vi "DC motor drive with k.vi"() -> ()   [LabVIEW 2019]
uses:
  <vilib>/addons/Control Design/_Model Construction/Data Typedefs.llb/CD Feedback Connections.ctl
  <vilib>/addons/Control Design/_Model Construction/Data Typedefs.llb/CD Root Locus with Gain Info.ctl
  <vilib>/addons/Control Design/_Model Construction/Model Creation.llb/Model Creation SubVI/cd_Create Transfer Function Model.vi
  <vilib>/addons/Control Design/_Utility/Model Viewer.llb/Model Viewer SubVI/cd_Draw Transfer Function Equation (TF).vi
  <vilib>/addons/Control Design/_Model Interconnection/Model Interconnection.llb/Model Interconnection SubVI/cd_Series (TF and TF).vi
  <vilib>/addons/Control Design/_Model Interconnection/Model Interconnection.llb/Model Interconnection SubVI/cd_Matrix Divide Models (TF and TF).vi
  <vilib>/addons/Control Design/_Model Interconnection/Model Interconnection.llb/Model Interconnection SubVI/cd_Feedback (TF and TF).vi
  <vilib>/addons/Control Design/_Model Construction/Special Model Creation.llb/Special Model Creation SubVI/CD Create PID Academic Model.vi
  <vilib>/addons/Control Design/_Model Interconnection/Model Interconnection.llb/Model Interconnection SubVI/cd_Unit Feedback (TF and TF).vi
  <vilib>/addons/Control Design/_Model Conversions/Model Type.llb/Model Conversion SubVI/cd_Convert Transfer Function to Zero-Pole-Gain Model.vi
  <vilib>/addons/Control Design/_Utility/Model Viewer.llb/Model Viewer SubVI/cd_Draw Zero-Pole-Gain Equation (ZPK).vi
  <vilib>/addons/Control Design/_Dynamic Analysis/Dynamic Analysis.llb/Dynamic Analysis subVI/cd_Pole-Zero Map (Transfer Function).vi
  <vilib>/addons/Control Design/_Dynamic Analysis/Dynamic Analysis.llb/Dynamic Analysis subVI/cd_Root Locus (Transfer Function).vi
  <vilib>/addons/Control Design/_Dynamic Analysis/Dynamic Analysis.llb/Dynamic Analysis subVI/cd_Stability (Transfer Function).vi
  <vilib>/addons/Control Design/_Model Construction/NI_LinSys_Model Creation.lvlib
  <vilib>/addons/Control Design/_Utility/NI_CD_Model Viewer.lvlib
  <vilib>/addons/Control Design/_Model Interconnection/NI_CD_Model Interconnection.lvlib
  <vilib>/addons/Control Design/_Dynamic Analysis/NI_CD_Dynamic Analysis.lvlib
  <vilib>/addons/Control Design/_Model Conversions/NI_CD_Model Type.lvlib
  <vilib>/addons/Control Design/_Model Construction/NI_CD_Special Model Creation.lvlib
  <vilib>/addons/Control Design/_Model Construction/NI_LinSys_Data Typedefs.lvlib
panel:
  out "Root Locus Information":T1
  out "Root Locus Graph":cluster{dbl[], dbl[]}[](graph)
  out "Stability":T2(ring)=enum."undetermined"
  out "G9(s)/(G7(s)":picture
  out "Zero-Pole-Gain Model":picture
  out "Overall transfer function":picture
  out "Zeros":cdb[](array[numeric]) format="%.4f"
  out "Poles":cdb[](array[numeric]) format="%.4f"
  out "Pole-Zero Map":cluster{dbl[], dbl[]}[](graph)
  in  "Feedback Connections":T3
  out "G10(s)":picture
  in  "Denominator 10":dbl[](array[numeric]) format="%#.5g"
  in  "Numerator 10":dbl[](array[numeric]) format="%#.5g"
  out "G9(s)":picture
  in  "Denominator 9":dbl[](array[numeric]) format="%#.5g"
  in  "Numerator 9":dbl[](array[numeric]) format="%#.5g"
  out "G8(s)":picture
  in  "Denominator 8":dbl[](array[numeric]) format="%#.5g"
  in  "Numerator 8":dbl[](array[numeric]) format="%#.5g"
  out "G7s)":picture
  in  "Denominator 7":dbl[](array[numeric]) format="%#.5g"
  in  "Numerator 7":dbl[](array[numeric]) format="%#.5g"
  out "G6(s)":picture
  in  "Denominator 6":dbl[](array[numeric]) format="%#.5g"
  in  "Numerator 6":dbl[](array[numeric]) format="%#.5g"
  out "G5(s)":picture
  in  "Denominator 5":dbl[](array[numeric]) format="%#.5g"
  in  "Numerator 5":dbl[](array[numeric]) format="%#.5g"
  out "G4(s)":picture
  in  "Denominator 4":dbl[](array[numeric]) format="%#.5g"
  in  "Numerator 4":dbl[](array[numeric]) format="%#.5g"
  out "G3(s)":picture
  in  "Denominator 3":dbl[](array[numeric]) format="%#.5g"
  in  "Numerator 3":dbl[](array[numeric]) format="%#.5g"
  out "G2(s)":picture
  in  "Denominator 2":dbl[](array[numeric]) format="%#.5g"
  in  "Numerator 2":dbl[](array[numeric]) format="%#.5g"
  out "G1(s)":picture
  in  "Denominator":dbl[](array[numeric]) format="%#.5g"
  in  "Numerator":dbl[](array[numeric]) format="%#.5g"
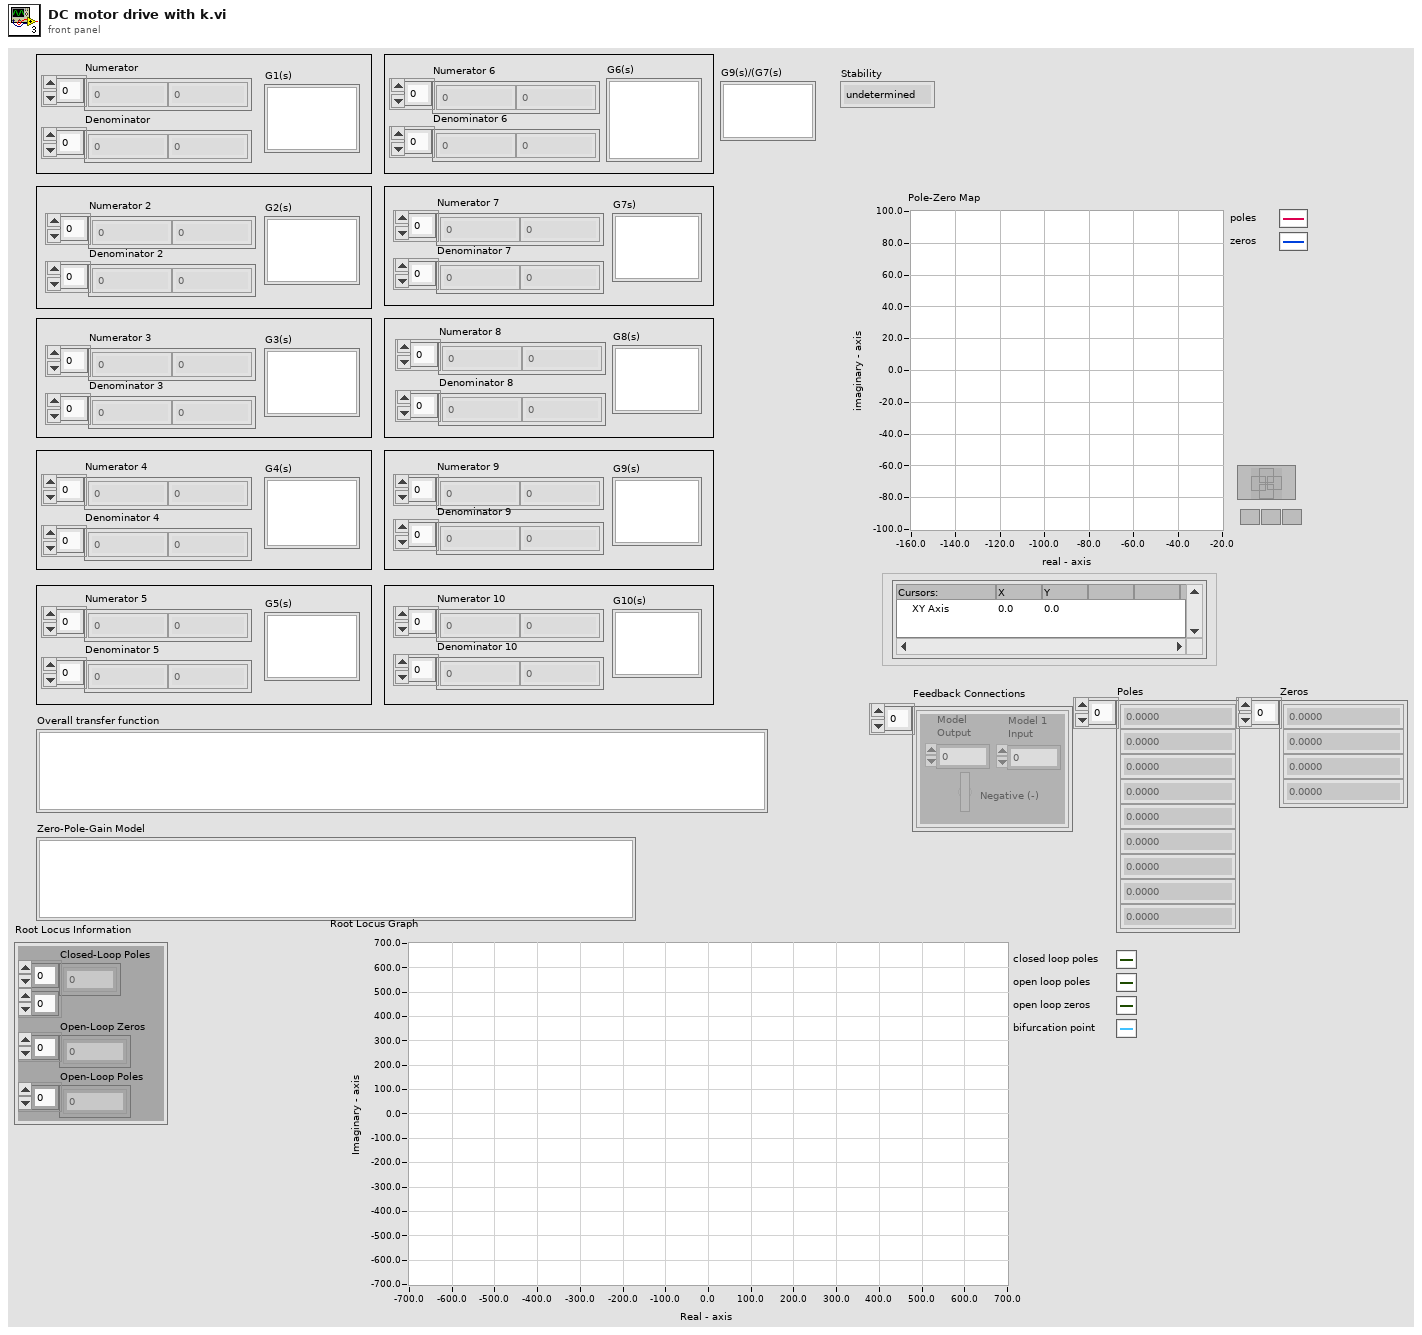
[diagram p1: front panel]
types:
  T1 = typedef "NI_LinSys_Data Typedefs.lvlib/CD Root Locus with Gain Info.ctl" = cluster{"Closed-Loop Poles":cdb[][], "Open-Loop Zeros":cdb[], "Open-Loop Poles":cdb[], "Bifurcation Points":cdb[], "K at Bifurcation Point":dbl[]}
  T2 = enum16{"stable", "marginally stable", "unstable", "undetermined"}
  T3 = typedef "NI_LinSys_Data Typedefs.lvlib/CD Feedback Connections.ctl" = cluster{"Model\nOutput":i32, "Model 1\nInput ":i32, "Signal":bool}[]
  T4 = typedef "NI_LinSys_Model Typedefs.lvlib/CD Transfer Function Model (MIMO).ctl" = cluster{"properties":T5, "transfer function(s)":T6[][]}
  T5 = typedef "NI_LinSys_Model Typedefs.lvlib/CD General Elements.ctl" = cluster{"Model name":string, "Input names":string[], "Output names":string[], "Input Delays":dbl[], "Output Delays":dbl[], "Sampling Time":dbl, "Notes":string}
  T6 = typedef "NI_LinSys_Model Typedefs.lvlib/CD Transfer Function Model (SISO).ctl" = cluster{"Numerator":dbl[], "Denominator":dbl[], "delay":dbl}
  T7 = typedef "NI_LinSys_Model Typedefs.lvlib/CD Zero-Pole-Gain Model (MIMO).ctl" = cluster{"properties":T5, "zero-pole-gain(s)":T8[][]}
  T8 = typedef "NI_LinSys_Model Typedefs.lvlib/CD Zero-Pole-Gain Model (SISO).ctl" = cluster{"Gain":dbl, "Zeros":cdb[], "Poles":cdb[], "delay":dbl}
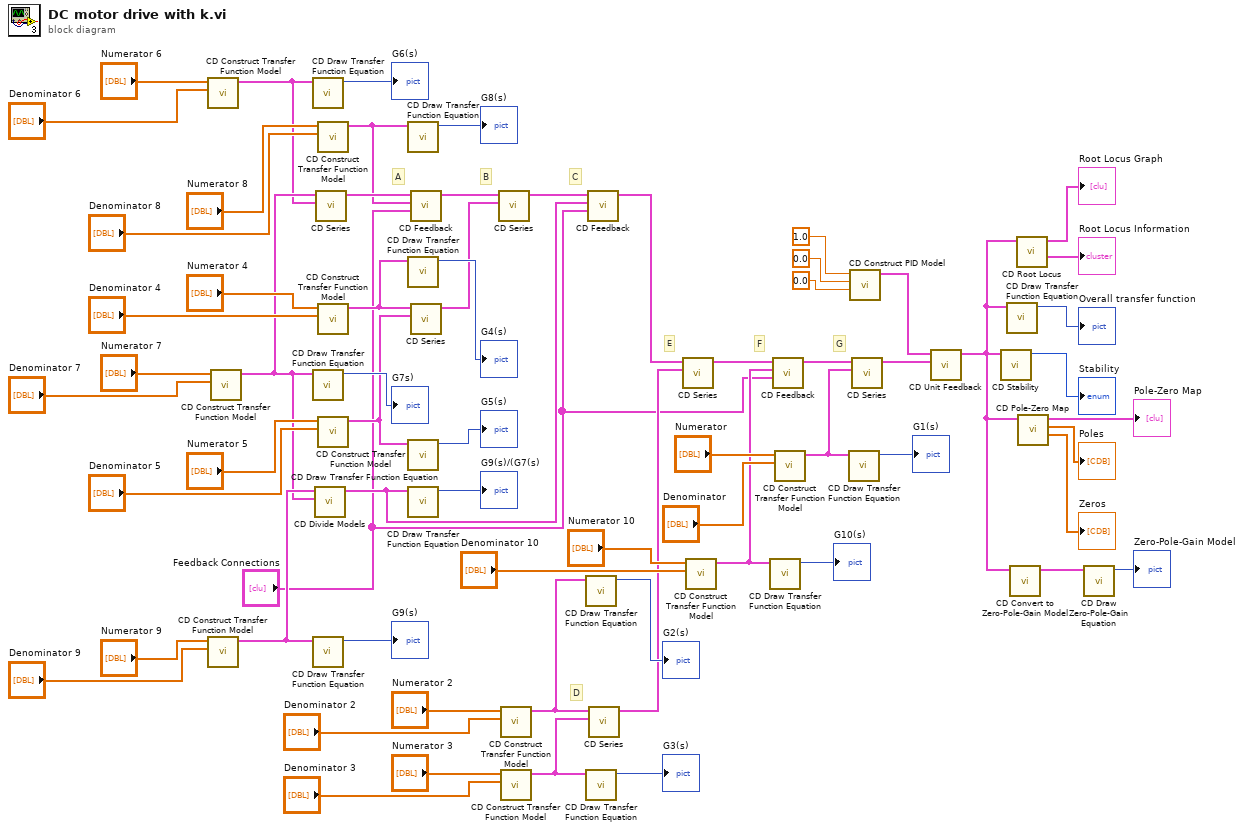
[diagram p0: block diagram]
diagram:
  # "G"
  # "F"
  # "E"
  # "D"
  # "C"
  # "B"
  # "A"
  n1 = call-poly <vilib>:"CD Construct Transfer Function Model.vi"("Denominator"="Denominator 6", "Numerator"="Numerator 6") -> ("Transfer Function Model"=w34:T4)  [unwired: 8 in, 1 out]
  n2 = call-poly <vilib>:"CD Construct Transfer Function Model.vi"("Denominator"="Denominator 9", "Numerator"="Numerator 9") -> ("Transfer Function Model"=w36:T4)  [unwired: 8 in, 1 out]
  n3 = call-poly <vilib>:"CD Construct Transfer Function Model.vi"("Denominator"="Denominator 7", "Numerator"="Numerator 7") -> ("Transfer Function Model"=w35:T4)  [unwired: 8 in, 1 out]
  n4 = call-poly <vilib>:"CD Draw Transfer Function Equation.vi"("Transfer Function Model"=w34) -> ("Equation"=→"G6(s)":picture)  [unwired: 8 in, 2 out]
  n5 = call-poly <vilib>:"CD Draw Transfer Function Equation.vi"("Transfer Function Model"=w35) -> ("Equation"=→"G7s)":picture)  [unwired: 8 in, 2 out]
  n6 = call-poly <vilib>:"CD Draw Transfer Function Equation.vi"("Transfer Function Model"=w36) -> ("Equation"=→"G9(s)":picture)  [unwired: 8 in, 2 out]
  n7 = call-poly <vilib>:"CD Divide Models.vi"("Model 2"=w35, "Model 1"=w36) -> ("Model Out"=w12:T4)  [unwired: 8 in, 1 out]
  n8 = call-poly <vilib>:"CD Series.vi"("Model 2"=w34, "Model 1"=w35) -> ("Series Model"=w33:T4)  [unwired: 8 in, 1 out]
  n9 = call-poly <vilib>:"CD Construct Transfer Function Model.vi"("Denominator"="Denominator 8", "Numerator"="Numerator 8") -> ("Transfer Function Model"=w32:T4)  [unwired: 8 in, 1 out]
  n10 = call-poly <vilib>:"CD Construct Transfer Function Model.vi"("Denominator"="Denominator 4", "Numerator"="Numerator 4") -> ("Transfer Function Model"=w29:T4)  [unwired: 8 in, 1 out]
  n11 = call-poly <vilib>:"CD Construct Transfer Function Model.vi"("Denominator"="Denominator 5", "Numerator"="Numerator 5") -> ("Transfer Function Model"=w28:T4)  [unwired: 8 in, 1 out]
  n12 = call-poly <vilib>:"CD Draw Transfer Function Equation.vi"("Transfer Function Model"=w32) -> ("Equation"=→"G8(s)":picture)  [unwired: 8 in, 2 out]
  n13 = call-poly <vilib>:"CD Draw Transfer Function Equation.vi"("Transfer Function Model"=w29) -> ("Equation"=→"G4(s)":picture)  [unwired: 8 in, 2 out]
  n14 = call-poly <vilib>:"CD Draw Transfer Function Equation.vi"("Transfer Function Model"=w28) -> ("Equation"=→"G5(s)":picture)  [unwired: 8 in, 2 out]
  n15 = call-poly <vilib>:"CD Draw Transfer Function Equation.vi"("Transfer Function Model"=w12) -> ("Equation"=→"G9(s)/(G7(s)":picture)  [unwired: 8 in, 2 out]
  n16 = call-poly <vilib>:"CD Feedback.vi"("Feedback Connections"="Feedback Connections", "Model 2"=w32, "Model 1"=w33) -> ("Closed-Loop Model"=w31:T4)  [unwired: 7 in, 1 out]
  n17 = call-poly <vilib>:"CD Series.vi"("Model 2"=w28, "Model 1"=w29) -> ("Series Model"=w30:T4)  [unwired: 8 in, 1 out]
  n18 = call-poly <vilib>:"CD Series.vi"("Model 2"=w30, "Model 1"=w31) -> ("Series Model"=w27:T4)  [unwired: 8 in, 1 out]
  n19 = call-poly <vilib>:"CD Construct Transfer Function Model.vi"("Denominator"="Denominator 2", "Numerator"="Numerator 2") -> ("Transfer Function Model"=w26:T4)  [unwired: 8 in, 1 out]
  n20 = call-poly <vilib>:"CD Construct Transfer Function Model.vi"("Denominator"="Denominator 3", "Numerator"="Numerator 3") -> ("Transfer Function Model"=w25:T4)  [unwired: 8 in, 1 out]
  n21 = call-poly <vilib>:"CD Draw Transfer Function Equation.vi"("Transfer Function Model"=w26) -> ("Equation"=→"G2(s)":picture)  [unwired: 8 in, 2 out]
  n22 = call-poly <vilib>:"CD Draw Transfer Function Equation.vi"("Transfer Function Model"=w25) -> ("Equation"=→"G3(s)":picture)  [unwired: 8 in, 2 out]
  n23 = call-poly <vilib>:"CD Feedback.vi"("Feedback Connections"="Feedback Connections", "Model 2"=w12, "Model 1"=w27) -> ("Closed-Loop Model"=w24:T4)  [unwired: 7 in, 1 out]
  n24 = call-poly <vilib>:"CD Series.vi"("Model 2"=w25, "Model 1"=w26) -> ("Series Model"=w23:T4)  [unwired: 8 in, 1 out]
  n25 = call-poly <vilib>:"CD Series.vi"("Model 2"=w23, "Model 1"=w24) -> ("Series Model"=w22:T4)  [unwired: 8 in, 1 out]
  n26 = call-poly <vilib>:"CD Construct Transfer Function Model.vi"("Denominator"="Denominator 10", "Numerator"="Numerator 10") -> ("Transfer Function Model"=w21:T4)  [unwired: 8 in, 1 out]
  n27 = call-poly <vilib>:"CD Draw Transfer Function Equation.vi"("Transfer Function Model"=w21) -> ("Equation"=→"G10(s)":picture)  [unwired: 8 in, 2 out]
  n28 = call-poly <vilib>:"CD Feedback.vi"("Feedback Connections"="Feedback Connections", "Model 2"=w21, "Model 1"=w22) -> ("Closed-Loop Model"=w20:T4)  [unwired: 7 in, 1 out]
  n29 = call-poly <vilib>:"CD Construct Transfer Function Model.vi"("Denominator"="Denominator", "Numerator"="Numerator") -> ("Transfer Function Model"=w19:T4)  [unwired: 8 in, 1 out]
  n30 = call-poly <vilib>:"CD Draw Transfer Function Equation.vi"("Transfer Function Model"=w19) -> ("Equation"=→"G1(s)":picture)  [unwired: 8 in, 2 out]
  n31 = call-poly <vilib>:"CD Construct PID Model.vi"("Derivative time [s] (Td)"=0.0, "Integral time [s] (Ti)"=0.0, "Proportional Gain (Kc)"=1.0) -> ("Transfer Function Model"=w6:T4)  [unwired: 7 in, 1 out]
  n32 = call-poly <vilib>:"CD Series.vi"("Model 2"=w19, "Model 1"=w20) -> ("Series Model"=w2:T4)  [unwired: 8 in, 1 out]
  n33 = call-poly <vilib>:"CD Unit Feedback.vi"("Model 2"=w2, "Model 1"=w6) -> ("Closed-Loop Model"=w1:T4)  [unwired: 8 in, 1 out]
  n34 = call-poly <vilib>:"CD Stability.vi"("Transfer Function Model"=w1) -> ("Stability"=→"Stability":T2)  [unwired: 8 in, 2 out]
  n35 = call-poly <vilib>:"CD Draw Transfer Function Equation.vi"("Transfer Function Model"=w1) -> ("Equation"=→"Overall transfer function":picture)  [unwired: 8 in, 2 out]
  n36 = call-poly <vilib>:"CD Convert to Zero-Pole-Gain Model.vi"("Transfer Function Model"=w1) -> ("Zero-Pole-Gain Model"=w14:T7)  [unwired: 9 in, 1 out]
  n37 = call-poly <vilib>:"CD Root Locus.vi"("Transfer Function Model"=w1) -> ("Root Locus Information"=→"Root Locus Information":T1, "Root Locus Graph"=→"Root Locus Graph":cluster{dbl[], dbl[]}[])  [unwired: 7 in, 2 out]
  n38 = call-poly <vilib>:"CD Pole-Zero Map.vi"("Transfer Function Model"=w1) -> ("Zeros"=→"Zeros":cdb[], "Poles"=→"Poles":cdb[], "Pole-Zero Map"=→"Pole-Zero Map":cluster{dbl[], dbl[]}[])  [unwired: 7 in, 1 out]
  n39 = call-poly <vilib>:"CD Draw Zero-Pole-Gain Equation.vi"("Zero-Pole-Gain Model"=w14) -> ("Equation"=→"Zero-Pole-Gain Model":picture)  [unwired: 8 in, 2 out]
